vi "Model_GetAttributes.vi"(8 "error in (no error)":errorcluster caption="错误输入（无错误）", 11 "User Management Model 输入":refnum<class "User Management Model.lvclass">) -> (0 "error out":errorcluster caption="错误输出", 1 "数据值":T1, 2 "属性引用":refnum<data-value>, 3 "User Management Model 输出":refnum<class "User Management Model.lvclass">)   [LabVIEW 2019, in "User Management Model.lvclass"]
uses:
  User Management Model.lvclass
  protect/ObjectAttributes.ctl
  User Management Model.lvclass/User Management Model.ctl
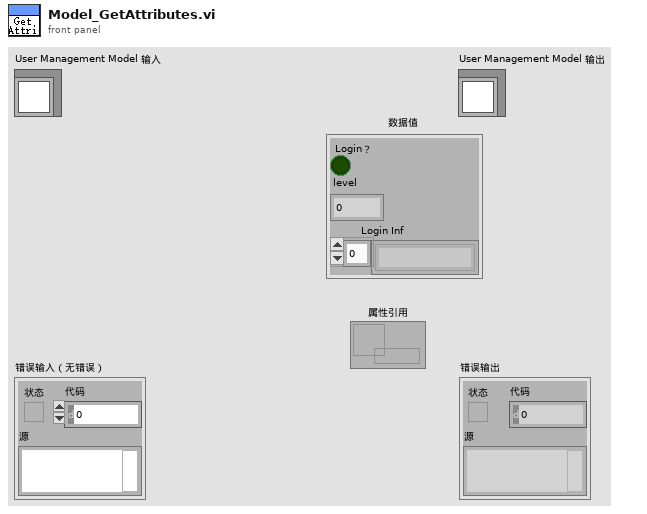
[diagram p1: front panel]
types:
  T1 = typedef "User Management Model.lvclass/ObjectAttributes.ctl" = cluster{"Login？":bool, "level":i32, "Login Inf":string[]}
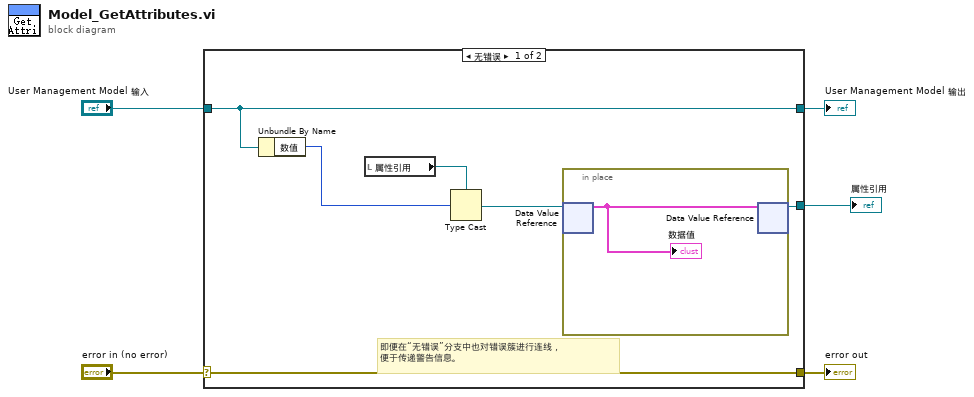
[diagram p0: block diagram]
diagram:
  n1 = case shown="无错误" "error in (no error)" {
    selector: "error in (no error)" -> [w11 w14]
    tunnel: [w11 w14] -> w4
    tunnel: [w10 w13] -> w2
    tunnel: "User Management Model 输入" -> [w10 w13]
    tunnel: [w6 _] -> w1
    frame No Error {
      # "即便在“无错误”分支中也对错误簇进行连线，\n便于传递警告信息。"
      n2 = Unbundle By Name(w10) -> ("数值"=w9:u32)
      n3 = local read "属性引用"() -> (w8:refnum<data-value>)
      n4 = Type Cast(type=w8, x=w9) -> (*(type *) &x=w7:refnum<data-value>)
      n5 = in-place {
        n6 = in-place-dvr #1(w7) -> (w12:T1)  [unwired: 1 out]
        "数据值" <- w12
        n7 = in-place-dvr #1(w12) -> (w6:refnum<data-value>)  [unwired: 1 out]
      }
    }
    frame Error {
    }
  }
  "error out" <- w4
  "User Management Model 输出" <- w2
  "属性引用" <- w1
